vi "Stats_SubVI.vi"(4 "Input Array":dbl[](array[numeric])) -> (0 "Std Dev":dbl, 1 "Mean":dbl, 2 "Max":dbl, 3 "Min":dbl)   [LabVIEW 2025]
uses:
  <vilib>/Analysis/baseanly.llb/Mean (DBL).vi
  <vilib>/Analysis/NI_AALBase.lvlib
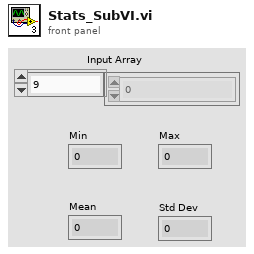
[diagram p1: front panel]
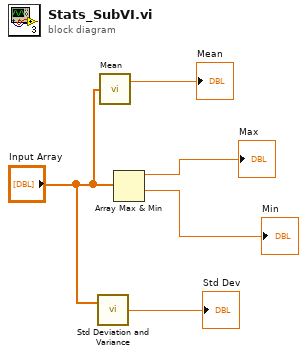
[diagram p0: block diagram]
diagram:
  n1 = call <vilib>:"Std Deviation and Variance.vi"("X"="Input Array") -> ("standard deviation"=→"Std Dev":dbl)  [unwired: 1 in, 2 out]
  n2 = call-poly <vilib>:"Mean.vi"("X"="Input Array") -> ("mean"=→"Mean":dbl)  [unwired: 1 out]
  n3 = Array Max & Min(array="Input Array") -> (max value=→"Max":dbl, min value=→"Min":dbl)  [unwired: 2 out]
